vi "GetSimulatedIMU.vi"(4 "Real IMU Yaw (deg)":dbl format="%#_13g", 5 "Rotation Command":dbl, 6 "Auto Test Mode":bool, 7 "Max Simulated Rotation Speed (deg/s)":dbl=180.0, 8 "Reset Yaw (deg)":dbl format="%#_13g", 11 "Reset Yaw":bool) -> (1 "Simulated Roll (deg)":dbl, 2 "Simulated Pitch (deg)":dbl, 3 "Simulated Yaw (deg)":dbl)   [LabVIEW 2019]
doc: "This VI simulates an IMU yaw reading based on the current drive base rotation command. It is intended for use when when testing autonomous plays on the robot cart. Pose pushes and resets are handled identically to the real IMU yaw sensor."
uses:
  <vilib>/Rock Robotics/WPI/DriverStation/WPI_DriverStationRobotMode2.ctl
  dsdata.vi
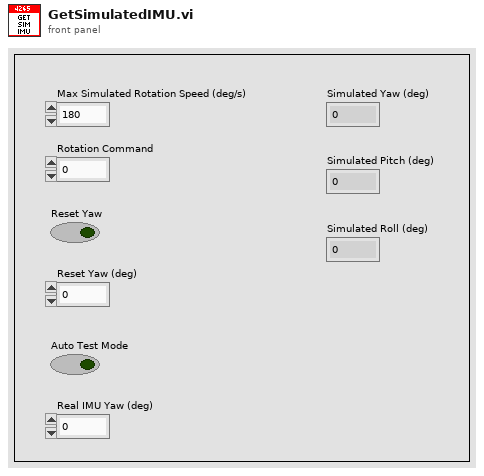
[diagram p1: front panel]
types:
  T1 = typedef "WPI_DriverStationRobotMode2.ctl" = enum16{"Autonomous Disabled", "Autonomous Enabled", "Teleop Disabled", "Teleop Enabled", "Disconnected", "Finish", "Test Disabled", "Test Enabled", "Emergency Stopped"}
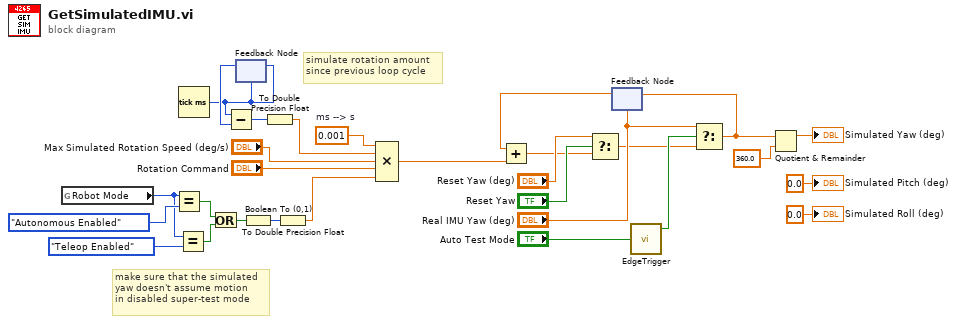
[diagram p0: block diagram]
diagram:
  w20 = 0.001  # ms --> s
  # "make sure that the simulated\nyaw doesn't assume motion\nin disabled super-test mode"
  # "simulate rotation amount\nsince previous loop cycle"
  n1 = global read "dsdata.vi" "Robot Mode"() -> (w9:T1)
  n2 = Equal?(x=w9, y=WPI_DriverStationRobotMode2."Autonomous Enabled") -> (x = y?=w6:bool)
  n3 = Equal?(x=w9, y=WPI_DriverStationRobotMode2."Teleop Enabled") -> (x = y?=w7:bool)
  n4 = Tick Count (ms)() -> (millisecond timer value=w16:u32)
  n5 = Or(x=w6, y=w7) -> (x .or. y?=w1:bool)
  n6 = feedback #1(w16) -> (w17:u32)
  n7 = Subtract(x=w16, y=w17) -> (x-y=w18:u32)
  n8 = feedback-in #1(w16) -> ()
  n9 = Boolean To (0,1)(Boolean=w1) -> (0, 1=w5:i16)
  n10 = To Double Precision Float(number=w18) -> (double precision float=w19:dbl)
  n11 = To Double Precision Float(number=w5) -> (double precision float=w4:dbl)
  n12 = Compound Arithmetic op=MULTIPLY(w20, w19, "Max Simulated Rotation Speed (deg/s)", "Rotation Command", w4) -> (w13:dbl)
  n13 = feedback #2("Real IMU Yaw (deg)") -> (w12:dbl)
  n14 = Add(x=w12, y=w13) -> (x+y=w21:dbl)
  n15 = Select(t="Reset Yaw (deg)", s="Reset Yaw", f=w21) -> (s? t:f=w22:dbl)
  n16 = call "EdgeTrigger.vi"("Input Signal"="Auto Test Mode") -> ("Rising Edge Trigger"=w27:bool)  [unwired: 2 out]
  n17 = Select(t="Real IMU Yaw (deg)", s=w27, f=w22) -> (s? t:f=w23:dbl)
  n18 = feedback-in #2(w23) -> ()
  n19 = Quotient & Remainder(x=w23, y=360.0) -> (x-y*floor(x/y)=→"Simulated Yaw (deg)":dbl)  [unwired: 1 out]
  "Simulated Pitch (deg)" <- 0.0 ("Simulated Pitch (deg)")
  "Simulated Roll (deg)" <- 0.0 ("Simulated Roll (deg)")
